vi "Read Base Actor Events.vi"(11 "Template in":refnum<class "Template.lvclass">) -> (3 "Base Actor Events":T1)   [LabVIEW 2020, in "Template.lvlib" / "Template.lvclass"]
uses:
  Template.lvclass
  typedefs/base actor events.ctl
  Template.lvclass/Template.ctl
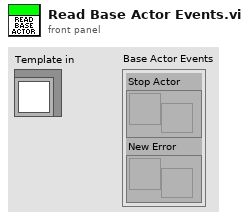
[diagram p1: front panel]
types:
  T1 = typedef "Template.lvlib/Template.lvclass/base actor events.ctl" = cluster{"Stop Actor":refnum<user-event>, "New Error":refnum<user-event>}
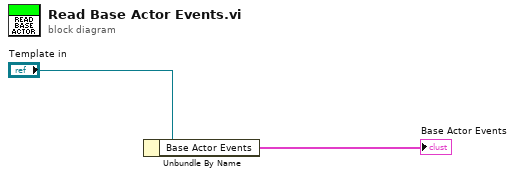
[diagram p0: block diagram]
diagram:
  n1 = Unbundle By Name("Template in") -> ("Base Actor Events"=→"Base Actor Events":T1)
